vi "PQgetTableNoTrans.vi"(8 "error in":errorcluster, 10 "query":string, 11 "conn":u32) -> (0 "error out":errorcluster, 1 "Data":string[][](array[string]), 3 "conn_out":u32, 4 "PQnFields":i32, 6 "PQnTuples":i32)   [LabVIEW 2019, in "libpqutility.lvlib"]
uses:
  libpqutility.lvlib
  libpqlv/src/PQnfields.vi
  libpqlv/src/PQntuples.vi
  libpqlv/src/PQgetvalue.vi
  libpqlv/libpqlv.lvlib
panel:
  out "PQsendQuery":i32
  out "PQresultStatus":T1(ring)
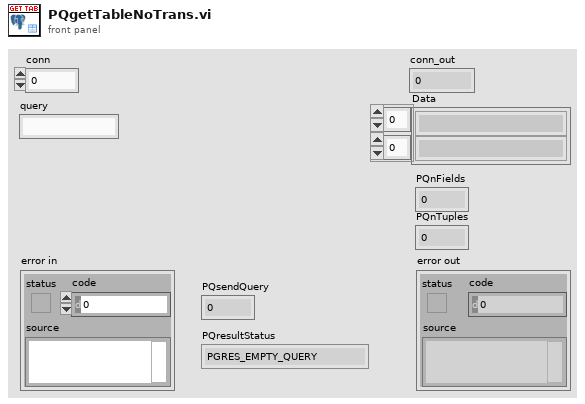
[diagram p1: front panel]
types:
  T1 = enum16{"PGRES_EMPTY_QUERY", "PGRES_COMMAND_OK", "PGRES_TUPLES_OK", "PGRES_COPY_OUT", "PGRES_COPY_IN", "PGRES_BAD_RESPONSE", "PGRES_NONFATAL_ERROR", "PGRES_FATAL_ERROR"}
  T2 = enum32{"PGRES_EMPTY_QUERY", "PGRES_COMMAND_OK", "PGRES_TUPLES_OK", "PGRES_COPY_OUT", "PGRES_COPY_IN", "PGRES_BAD_RESPONSE", "PGRES_NONFATAL_ERROR", "PGRES_FATAL_ERROR"}
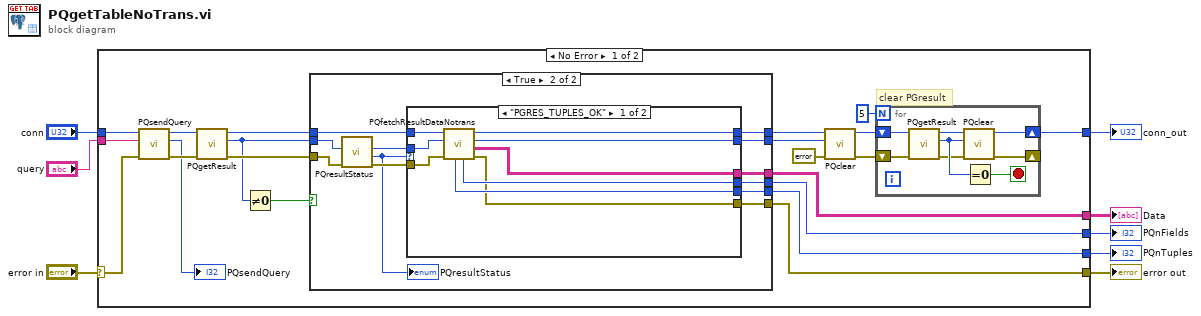
[diagram p0: block diagram]
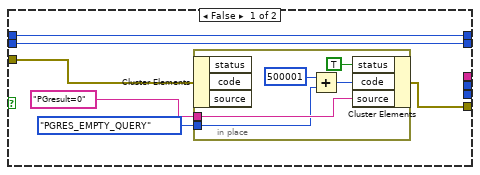
[diagram p2: hidden frame]
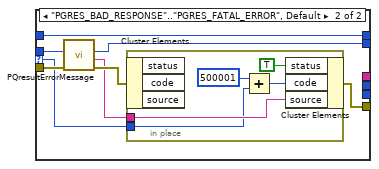
[diagram p3: hidden frame]
diagram:
  n1 = case shown="No Error" "error in" {
    selector: "error in" -> [w28 w84]
    tunnel: "conn" -> [w22 w83]
    tunnel: [w29 w84] -> w7
    tunnel: [w10 w83] -> w5
    tunnel: [w27 _] -> w4
    tunnel: "query" -> [w25 _]
    tunnel: [w24 _] -> w2
    tunnel: [w23 _] -> w1
    frame No Error {
      # "clear PGresult"
      n2 = call "PQsendQuery.vi"("error in (no error)"=w28, "query"=w25, "conn"=w22) -> ("error out"=w21:errorcluster, "PQsendQuery"=→"PQsendQuery":i32, "conn_out"=w14:u32)  [unwired: 6 in]
      n3 = call "PQgetResult.vi"("error in (no error)"=w21, "conn"=w14) -> ("error out"=w20:errorcluster, "PGresult"=w19:u32, "conn_out"=w13:u32)  [unwired: 7 in]
      n4 = Not Equal To 0?(x=w19) -> (x != 0?=w18:bool)
      n5 = case shown="True" w18 {
        tunnel: w20 -> [w31 w52]
        tunnel: w13 -> [w34 w51]
        tunnel: [_ w49] -> w27
        tunnel: [_ w48] -> w24
        tunnel: [w30 w47] -> w29
        tunnel: w19 -> [w35 w45]
        tunnel: [_ w46] -> w23
        tunnel: [w35 w43] -> w15
        tunnel: [w34 w41] -> w12
        frame False {
          n6 = in-place {
            in-place-border: "PGresult=0" ("source") -> [w40]
            in-place-border: T2."PGRES_EMPTY_QUERY" ("PQresultStatus") -> [w37]
            n7 = in-place-cluster #1(w31) -> ()  [unwired: 3 out]
            n8 = Add(x=u32 500001, y=w37) -> (x+y=w36:u32)
            n9 = in-place-cluster #1("status"=TRUE, "code"=w36, "source"=w40) -> (w30:errorcluster)
          }
        }
        frame True {
          n10 = call "PQresultStatus.vi"("error in (no error)"=w52, "res"=w45) -> ("error out"=w50:errorcluster, "PQresultStatus"=w44:T2, "res out"=w42:u32)  [unwired: 7 in]
          "PQresultStatus" <- w44
          n11 = case shown="\"PGRES_TUPLES_OK\"" w44 {
            selector: w44 -> [_ w63]
            tunnel: w42 -> [w59 w67]
            tunnel: [w54 _] -> w48
            tunnel: w50 -> [w56 w69]
            tunnel: w51 -> [w60 w68]
            tunnel: [w57 _] -> w49
            tunnel: [w53 w62] -> w47
            tunnel: [w55 _] -> w46
            tunnel: [w58 w64] -> w43
            tunnel: [w61 w68] -> w41
            frame "PGRES_TUPLES_OK" {
              n12 = call "PQfetchResultDataNotrans.vi"("error in"=w56, "res"=w59, "conn"=w60) -> ("error out"=w53:errorcluster, "Data"=w57:string[][], "res_out"=w58:u32, "conn_out"=w61:u32, "PQnFields"=w54:i32, "PQnTuples"=w55:i32)  [unwired: 3 in]
            }
            frame "PGRES_BAD_RESPONSE".."PGRES_FATAL_ERROR", Default {
              n13 = call "PQresultErrorMessage.vi"("error in (no error)"=w69, "res"=w67) -> ("error out"=w66:errorcluster, "PQresultErrorMessage"=w65:string, "res out"=w64:u32)  [unwired: 7 in]
              n14 = in-place {
                in-place-border: w65 -> [w74]
                in-place-border: w63 -> [w71]
                n15 = in-place-cluster #2(w66) -> ()  [unwired: 3 out]
                n16 = Add(x=u32 500001, y=w71) -> (x+y=w70:u32)
                n17 = in-place-cluster #2("status"=TRUE, "code"=w70, "source"=w74) -> (w62:errorcluster)
              }
            }
          }
        }
      }
      n18 = call "PQclear.vi"("error in (no error)"=errorcluster {"status"=FALSE, "code"=0, "source"=""}, "res"=w15, "conn"=w12) -> ("error out"=w11:errorcluster, "conn_out"=w26:u32)  [unwired: 7 in]
      n19 = for {
        N: 5 -> [_]
        shift-right: [w75] -> _
        shift-left: w11 -> [w78]
        shift-right: [w77] -> w10
        shift-left: w26 -> [w79]
        stop <- w81 stop-if-true
        n20 = call "PQgetResult.vi"("error in (no error)"=w78, "conn"=w79) -> ("error out"=w76:errorcluster, "PGresult"=w80:u32, "conn_out"=w82:u32)  [unwired: 7 in]
        n21 = call "PQclear.vi"("error in (no error)"=w76, "res"=w80, "conn"=w82) -> ("error out"=w75:errorcluster, "conn_out"=w77:u32)  [unwired: 7 in]
        n22 = Equal To 0?(x=w80) -> (x = 0?=w81:bool)
      }
    }
    frame Error {
    }
  }
  "conn_out" <- w5
  "error out" <- w7
  "Data" <- w4
  "PQnFields" <- w2
  "PQnTuples" <- w1
